vi "UI Panels - Set Menu Items.vi"(6 "Menu":string[](array[string]), 7 "index":i32, 8 "error in (no error)":errorcluster, 11 "Panels_XControl In":refnum<vi>) -> (0 "error out":errorcluster, 3 "Panels_XControl Out":refnum<vi>)   [LabVIEW 2013, in "UI Panels.lvlib"]
uses:
  UI Panels.lvlib
  Panels_XControl.xctl
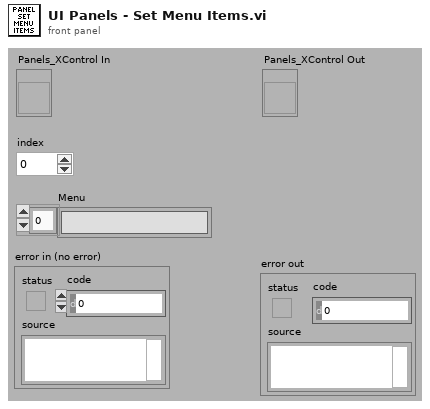
[diagram p1: front panel]
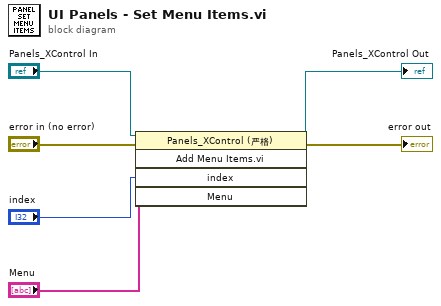
[diagram p0: block diagram]
diagram:
  n1 = invoke class="Panels_XControl (严格)" method="Add Menu Items.vi"(reference="Panels_XControl In", error in="error in (no error)", "index"="index", "Menu"="Menu") -> (reference out=→"Panels_XControl Out":refnum<vi>, error out=→"error out":errorcluster)  [unwired: 1 in, 3 out]
